vi "GetAxisExtendedDataResults.vi"(6 "argument":i32, 7 "axisExtendedIndex":i32, 8 "error in (no error)":errorcluster, 9 "axis extended data signal":u32(ring)=10 items=["AmplifierPeakCurrent"=303, "AmplifierTemperature"=309, "AnalogInput0"=10, "AnalogInput1"=11, "AnalogInput2"=28, "AnalogInput3"=29, "AnalogOutput0"=36, "AnalogOutput1"=37, "AnalogOutput2"=38, "AnalogOutput3"=39, "AnalogSensorInput"=446, "BoardRevision"=407, "BusVoltage"=375, "BusVoltageNegative"=441, "CapacitanceSensorRawPosition"=415, "CommandOutputType"=389, "ControlEffort"=282, "CurrentCommand"=8, "CurrentFeedback"=7, "DataAcquisitionSamples"=234, "DriveFeedforwardOutput"=404, "DriveMemoryDouble"=42, "DriveMemoryDoublePointer"=206, "DriveMemoryFloat"=41, "DriveMemoryFloatPointer"=205, "DriveMemoryInt16"=157, "DriveMemoryInt16Pointer"=203, "DriveMemoryInt32"=40, "DriveMemoryInt32Pointer"=202, "DriveMemoryInt8"=158, "DriveMemoryInt8Pointer"=204, "DriveTimer"=44, "DriveTimerMax"=319, "DriveTypeID"=305, "EncoderCosine"=27, "EncoderSine"=26, "EnDatAbsolutePosition"=269, "EthernetDebuggingInformation"=365, "FaultPositionFeedback"=372, "FirmwareRevision"=408, "FirmwareVersionBuild"=318, "FirmwareVersionMajor"=315, "FirmwareVersionMinor"=316, "FirmwareVersionPatch"=317, "FPGAVersion"=304, "GalvoLaserOutput"=409, "GalvoLaserPowerCorrectionOutput"=414, "InternalErrorCode"=314, "IOBoardInstalled"=374, "LastTickCounter"=405, "LatchedMarkerPosition"=331, "LoopTransmissionAfter"=31, "LoopTransmissionBefore"=30, "MarkerSearchDistance"=320, "MaximumVoltage"=388, "ModbusBitMasterInputBits"=290, "ModbusBitMasterOutputBits"=291, "ModbusRegDoubleMasterInputWords"=298, "ModbusRegDoubleMasterOutputWords"=299, "ModbusRegInt16MasterInputWords"=292, "ModbusRegInt16MasterOutputWords"=293, "ModbusRegInt32MasterInputWords"=294, "ModbusRegInt32MasterOutputWords"=295, "ModbusRegSingleMasterInputWords"=296, "ModbusRegSingleMasterOutputWords"=297, "MotorCommutationAngle"=373, "MotorTemperature"=447, "MXAbsolutePosition"=311, "NpaqSyncoutStatus"=366, "PhaseACurrentFeedback"=24, "PhaseAVoltageCommand"=300, "PhaseBCurrentFeedback"=25, "PhaseBVoltageCommand"=301, "PhaseCVoltageCommand"=302, "PiezoVoltageCommand"=376, "PiezoVoltageFeedback"=377, "PositionCalibrationGalvo"=419, "PositionCommandDrive"=98, "PositionCommandGalvo"=237, "PositionDetectorVoltage"=235, "PositionFeedbackDrive"=88, "PositionFeedbackGalvo"=327, "ProcessorTemperature"=442, "PSOBitArrayIndex"=310, "PSOCounter1"=229, "PSOCounter2"=230, "PSOCounter3"=231, "PSODistanceArrayIndex"=308, "PSOStatus"=43, "PSOWindow1"=232, "PSOWindow1ArrayIndex"=306, "PSOWindow2"=233, "PSOWindow2ArrayIndex"=307, "ResoluteAbsolutePosition"=369, "ResoluteStatus"=449, "ResolverChannel1"=267, "ResolverChannel2"=268, "ServoUpdateRate"=312, "SettlingTime"=313, "STOStatus"=443, "TemperatureSensor"=332, "TimeSinceReset"=387, "ZHSDifference"=32, "ZHSFiltered"=35, "ZHSSum"=33, "ZHSUnfiltered"=34], 10 "Data In":refnum<k24>, 11 "controller in":refnum<k24>) -> (0 "error out":errorcluster, 1 "AxisExtendedData":dbl[](array[numeric]), 2 "Data Out":refnum<k24>, 3 "controller out":refnum<k24>)   [LabVIEW 2018, in "Aerotech.lvlib"]
uses:
  Aerotech.lvlib
  C:/Users/HEP/Documents/GitHub/UCSB-Gantry-HEP-2018/Drivers/Aerotech A3200/Bin/Aerotech.A3200.LabVIEW.dll
  UCSB-Gantry-HEP-2018/Drivers/Aerotech A3200/Bin/Aerotech.A3200.LabVIEW.dll
  C:/Program Files (x86)/Aerotech/A3200/LabVIEW/2010/Bin/Aerotech.A3200.dll
  Program Files (x86)/Aerotech/A3200/LabVIEW/2010/Bin/Aerotech.A3200.dll
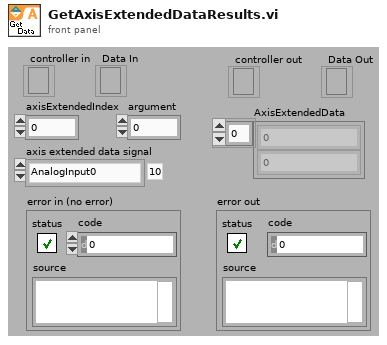
[diagram p1: front panel]
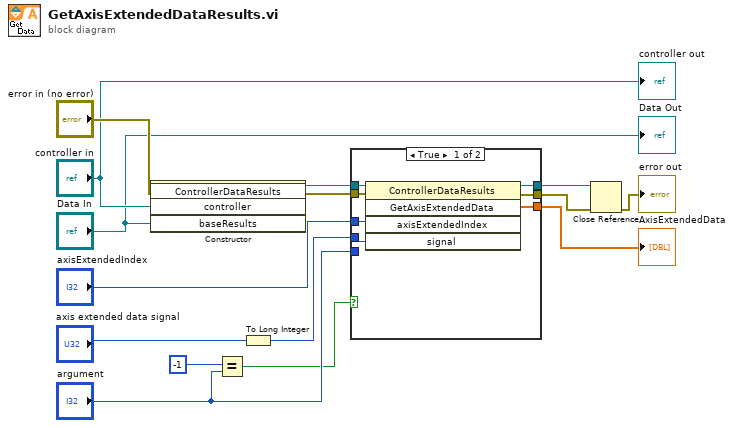
[diagram p0: block diagram]
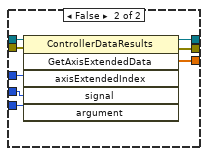
[diagram p2: hidden frame]
diagram:
  n1 = constructor class="ControllerDataResults"(error in="error in (no error)", "controller"="controller in", "baseResults"="Data In") -> (reference out=w14:refnum<k24>, error out=w13:errorcluster)  [unwired: 2 in, 3 out]
  n2 = Equal?(x=-1, y="argument") -> (x = y?=w5:bool)
  n3 = To Long Integer(number="axis extended data signal") -> (32bit integer=w4:i32)
  n4 = case shown="True" w5 {
    tunnel: "axisExtendedIndex" -> [w22 w30]
    tunnel: [w21 w29] -> w3
    tunnel: [w20 w28] -> w2
    tunnel: w14 -> [w19 w27]
    tunnel: w13 -> [w18 w26]
    tunnel: "argument" -> [_ w23]
    tunnel: [w17 w25] -> w12
    tunnel: w4 -> [w16 w24]
    frame True {
      n5 = invoke class="ControllerDataResults" method="GetAxisExtendedData"(reference=w19, error in=w18, "axisExtendedIndex"=w22, "signal"=w16) -> (reference out=w20:refnum<k24>, error out=w21:errorcluster, "GetAxisExtendedData"=w17:dbl[])  [unwired: 1 in, 2 out]
    }
    frame False {
      n6 = invoke class="ControllerDataResults" method="GetAxisExtendedData"(reference=w27, error in=w26, "axisExtendedIndex"=w30, "signal"=w24, "argument"=w23) -> (reference out=w28:refnum<k24>, error out=w29:errorcluster, "GetAxisExtendedData"=w25:dbl[])  [unwired: 1 in, 3 out]
    }
  }
  "AxisExtendedData" <- w12
  n7 = Close Reference(reference=w2, error in (no error)=w3) -> (error out=→"error out":errorcluster)
  "controller out" <- "controller in"
  "Data Out" <- "Data In"
